vi "Create Diagnostics Addon From Configuration.vi"(7 "Merge Path (.dat)":path, 8 "error in (no error)":errorcluster, 10 "Configuration":T1 {"DID Outputs"."Frames"."Signals"."Byte Order" items=["Little Endian", "Big Endian"]; "DID Outputs"."Frames"."Signals"."Data Type" items=["Signed", "Unsigned", "IEEE Float"]; "Memory Inputs"."Frames"."Signals"."Byte Order" items=["Little Endian", "Big Endian"]; "Memory Inputs"."Frames"."Signals"."Data Type" items=["Signed", "Unsigned", "IEEE Float"]; "Memory Outputs"."Frames"."Signals"."Byte Order" items=["Little Endian", "Big Endian"]; "Memory Outputs"."Frames"."Signals"."Data Type" items=["Signed", "Unsigned", "IEEE Float"]; "Routines"."Routine Array"."Stop Parameters"."Response"."Byte Order" items=["Little Endian", "Big Endian"]; "Routines"."Routine Array"."Stop Parameters"."Response"."Data Type" items=["Signed", "Unsigned", "IEEE Float"]; "Routines"."Routine Array"."Stop Parameters"."Cmd"."Byte Order" items=["Little Endian", "Big Endian"]; "Routines"."Routine Array"."Stop Parameters"."Cmd"."Data Type" items=["Signed", "Unsigned", "IEEE Float"]; "Routines"."Routine Array"."Request Parameters"."Response"."Byte Order" items=["Little Endian", "Big Endian"]; "Routines"."Routine Array"."Request Parameters"."Response"."Data Type" items=["Signed", "Unsigned", "IEEE Float"]; "Routines"."Routine Array"."Request Parameters"."Cmd"."Byte Order" items=["Little Endian", "Big Endian"]; "Routines"."Routine Array"."Request Parameters"."Cmd"."Data Type" items=["Signed", "Unsigned", "IEEE Float"]; "Routines"."Routine Array"."Start Parameters"."Response"."Byte Order" items=["Little Endian", "Big Endian"]; "Routines"."Routine Array"."Start Parameters"."Response"."Data Type" items=["Signed", "Unsigned", "IEEE Float"]; "Routines"."Routine Array"."Start Parameters"."Cmd"."Byte Order" items=["Little Endian", "Big Endian"]; "Routines"."Routine Array"."Start Parameters"."Cmd"."Data Type" items=["Signed", "Unsigned", "IEEE Float"]; "IO Controls"."IO Control Array"."Signals"."Response"."Byte Order" items=["Little Endian", "Big Endian"]; "IO Controls"."IO Control Array"."Signals"."Response"."Data Type" items=["Signed", "Unsigned", "IEEE Float"]; "IO Controls"."IO Control Array"."Signals"."Cmd"."Byte Order" items=["Little Endian", "Big Endian"]; "IO Controls"."IO Control Array"."Signals"."Cmd"."Data Type" items=["Signed", "Unsigned", "IEEE Float"]; "DTC"."DTC Control"."Signals"."Byte Order" items=["Little Endian", "Big Endian"]; "DTC"."DTC Control"."Signals"."Data Type" items=["Signed", "Unsigned", "IEEE Float"]; "Diagnostics Basic Configuraiton"."IO Mode" items=["CAN 2.0", "CAN FD", "CAN FD+BRS"]; "Diagnostics Basic Configuraiton"."Fill Byte" format="%.0x"; "Diagnostics Basic Configuraiton"."VW TP Channel ID" format="%.0x"; "Diagnostics Basic Configuraiton"."Receive UUDT ID" format="%.0x"; "Diagnostics Basic Configuraiton"."Receive Extension" format="%.0x"; "Diagnostics Basic Configuraiton"."Transmit Extension" format="%.0x"; "Diagnostics Basic Configuraiton"."Receive ID" format="%.0x"; "Diagnostics Basic Configuraiton"."Transmit ID" format="%.0x"; "DID Inputs"."Frames"."Signals"."Byte Order" items=["Little Endian", "Big Endian"]; "DID Inputs"."Frames"."Signals"."Data Type" items=["Signed", "Unsigned", "IEEE Float"]; "PID Inputs"."Frames"."Signals"."Byte Order" items=["Little Endian", "Big Endian"]; "PID Inputs"."Frames"."Signals"."Data Type" items=["Signed", "Unsigned", "IEEE Float"]; "PID Outputs"."Frames"."Signals"."Byte Order" items=["Little Endian", "Big Endian"]; "PID Outputs"."Frames"."Signals"."Data Type" items=["Signed", "Unsigned", "IEEE Float"]}, 11 "Custom Devices Ref":refnum<k24>) -> (0 "error out":errorcluster, 3 "Custom Devices Ref":refnum<k24>)   [LabVIEW 2019, in "Diagnostics Addon SysDef API.lvlib"]
uses:
  Diagnostics Addon SysDef API.lvlib
  System Explorer/Types/SysDef.Export.ctl
  Shared/Types/CAN.ctl
  Shared/Types/CAN.Interface.ctl
  Shared/Types/Protocol.ctl
  Shared/Types/Transport.ctl
  Shared/Types/Security.ctl
  Shared/Types/Security.Type.ctl
  System Explorer/Types/Frames.Export.ctl
  System Explorer/Types/Frame.Export.ctl
  Shared/Types/Signal.ctl
  System Explorer/Types/DPIDs.Export.ctl
  System Explorer/Types/DPID.Export.ctl
  Shared/Types/DPID.ctl
  Shared/Types/DPID.Rate.ctl
  System Explorer/Types/DTC.Export.ctl
  Shared/Types/DTC.Settings.ctl
  Shared/Types/DTC.Descriptor.ctl
  System Explorer/Types/DTCControl.Export.ctl
  Shared/Types/986x.ctl
  System Explorer/Types/Command.Export.ctl
  System Explorer/Types/Status.Export.ctl
  System Explorer/Types/IOControls.Export.ctl
  System Explorer/Types/IO.Export.ctl
  System Explorer/Types/CmdResp.Export.ctl
  System Explorer/Types/Routines.Export.ctl
  System Explorer/Types/Routine.Export.ctl
  System Explorer/Types/UserDefined.Export.ctl
  System Explorer/Types/UserDefined.Group.Export.ctl
  System Explorer/Types/UserDefined.Group.Message.Export.ctl
  NationalInstruments.VeriStand.SystemDefinitionAPI
  NationalInstruments.VeriStand.SystemStorage
  Shared/SubVIs/Constants.vi
  Shared/Diagnostics Addon Shared.lvlib
  System Explorer/Diagnostics Addon System Explorer.lvlib
  <vilib>/NI/NI VeriStand Custom Device Import and Export Tool/ImportExport.lvlib
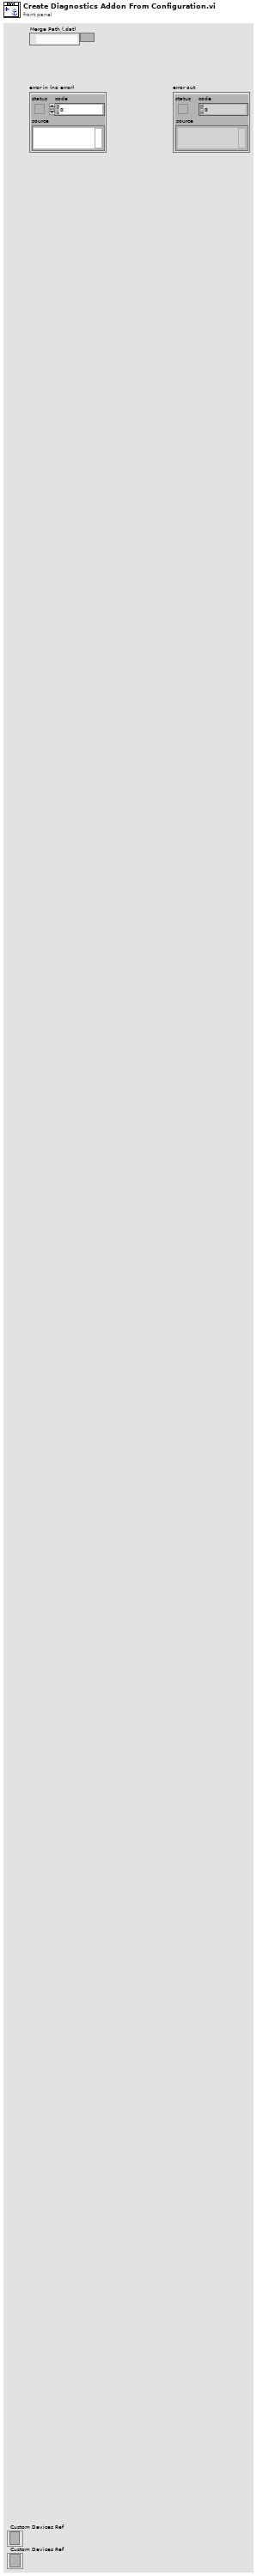
[diagram p1: front panel]
types:
  T1 = typedef "Diagnostics Addon System Explorer.lvlib/SysDef.Export.ctl" = cluster{"Name":string, "Description":string, "Diagnostics Basic Configuraiton":T2, "DID Outputs":T8, "DID Inputs":T8, "PID Outputs":T8, "PID Inputs":T8, "DPIDs":T11, "DTC":T15, "NI 986x Support":T19, "Commands":T20, "Status":T21, "IO Controls":T22, "Routines":T25, "Memory Outputs":T8, "Memory Inputs":T8, "User Defined":T27}
  T2 = typedef "Diagnostics Addon Shared.lvlib/CAN.ctl" = cluster{"Interface":T3, "Baud Rate":u64, "Diagnostic Protocol":T4, "Transport Protocol":T5, "Transmit ID":u32, "Receive ID":u32, "Transmit Extension":u8, "Receive Extension":u8, "Receive UUDT ID":u32, "Enable Stream":bool, "VW TP Channel ID":u32, "Fill Frame":bool, "Fill Byte":u8, "Termination":bool, "LIN Cluster":refnum<k21>, "NAD":u8, "IO Mode":u32, "Max DLC":u16, "FD Baud Rate":u64, "Security":T6}
  T3 = typedef "Diagnostics Addon Shared.lvlib/CAN.Interface.ctl" = string
  T4 = typedef "Diagnostics Addon Shared.lvlib/Protocol.ctl" = enum16{"GMLAN", "KWP-2000", "UDS", "User-Defined"}
  T5 = typedef "Diagnostics Addon Shared.lvlib/Transport.ctl" = enum16{"ISO TP - Normal Mode", "ISO TP - Mixed Mode", "VW TP 2.0", "Diagnostics on IP", "ISO TP LIN"}
  T6 = typedef "Diagnostics Addon Shared.lvlib/Security.ctl" = cluster{"Type":T7, "Source DLL Path":path, "Target DLL Path":path, "Security Level":u8, "Master Key":string}
  T7 = typedef "Diagnostics Addon Shared.lvlib/Security.Type.ctl" = enum16{"None", "DLL", "MasterKey"}
  T8 = typedef "Diagnostics Addon System Explorer.lvlib/Frames.Export.ctl" = cluster{"Description":string, "Frames":T9[]}
  T9 = typedef "Diagnostics Addon System Explorer.lvlib/Frame.Export.ctl" = cluster{"Name":string, "Description":string, "ID":u32, "Signals":T10[]}
  T10 = typedef "Diagnostics Addon Shared.lvlib/Signal.ctl" = cluster{"Start Bit":u32, "Length":u32, "Scaling Factor":dbl, "Scaling Offset":dbl, "Minimum":dbl, "Maximum":dbl, "Data Type":u32, "Byte Order":u32, "Default Value":dbl, "Name":string, "Units":string, "Description":string}
  T11 = typedef "Diagnostics Addon System Explorer.lvlib/DPIDs.Export.ctl" = cluster{"Description":string, "DPIDs":T12[]}
  T12 = typedef "Diagnostics Addon System Explorer.lvlib/DPID.Export.ctl" = cluster{"Name":string, "Description":string, "DPID":T13}
  T13 = typedef "Diagnostics Addon Shared.lvlib/DPID.ctl" = cluster{"DPID ID":u8, "Speed":T14, "PIDs":u16[]}
  T14 = typedef "Diagnostics Addon Shared.lvlib/DPID.Rate.ctl" = enum16{"Slow", "Medium", "Fast"}
  T15 = typedef "Diagnostics Addon System Explorer.lvlib/DTC.Export.ctl" = cluster{"Description":string, "Settings":T16, "DTC Control":T18, "Created DTCs":u32}
  T16 = typedef "Diagnostics Addon Shared.lvlib/DTC.Settings.ctl" = cluster{"Descriptor":T17, "Value.Code":dbl[], "Value.String":string[], "Value.J2012String":string[], "Status.Code":dbl[], "Status.String":string[]}
  T17 = typedef "Diagnostics Addon Shared.lvlib/DTC.Descriptor.ctl" = cluster{"DTC Byte Length":i32, "Status Byte Length":i32, "Add Data Byte Length":i32, "Byte Order":enum16{"Motorola", "Intel"}}
  T18 = typedef "Diagnostics Addon System Explorer.lvlib/DTCControl.Export.ctl" = cluster{"Description":string, "Signals":T10[]}
  T19 = typedef "Diagnostics Addon Shared.lvlib/986x.ctl" = cluster{"Enable":bool, "RIO Device":string, "Bitfile":path}
  T20 = typedef "Diagnostics Addon System Explorer.lvlib/Command.Export.ctl" = cluster{"Description":string}
  T21 = typedef "Diagnostics Addon System Explorer.lvlib/Status.Export.ctl" = cluster{"Description":string}
  T22 = typedef "Diagnostics Addon System Explorer.lvlib/IOControls.Export.ctl" = cluster{"Description":string, "IO Control Array":T23[]}
  T23 = typedef "Diagnostics Addon System Explorer.lvlib/IO.Export.ctl" = cluster{"Name":string, "Description":string, "ID":u16, "Signals":T24}
  T24 = typedef "Diagnostics Addon System Explorer.lvlib/CmdResp.Export.ctl" = cluster{"Cmd":T10[], "Response":T10[]}
  T25 = typedef "Diagnostics Addon System Explorer.lvlib/Routines.Export.ctl" = cluster{"Description":string, "Routine Array":T26[]}
  T26 = typedef "Diagnostics Addon System Explorer.lvlib/Routine.Export.ctl" = cluster{"Name":string, "Description":string, "ID":u16, "Start Parameters":T24, "Request Parameters":T24, "Stop Parameters":T24}
  T27 = typedef "Diagnostics Addon System Explorer.lvlib/UserDefined.Export.ctl" = cluster{"Description":string, "Groups":T28[]}
  T28 = typedef "Diagnostics Addon System Explorer.lvlib/UserDefined.Group.Export.ctl" = cluster{"Name":string, "Description":string, "Messages":T29[]}
  T29 = typedef "Diagnostics Addon System Explorer.lvlib/UserDefined.Group.Message.Export.ctl" = cluster{"Name":string, "Description":string, "Signals":T24}
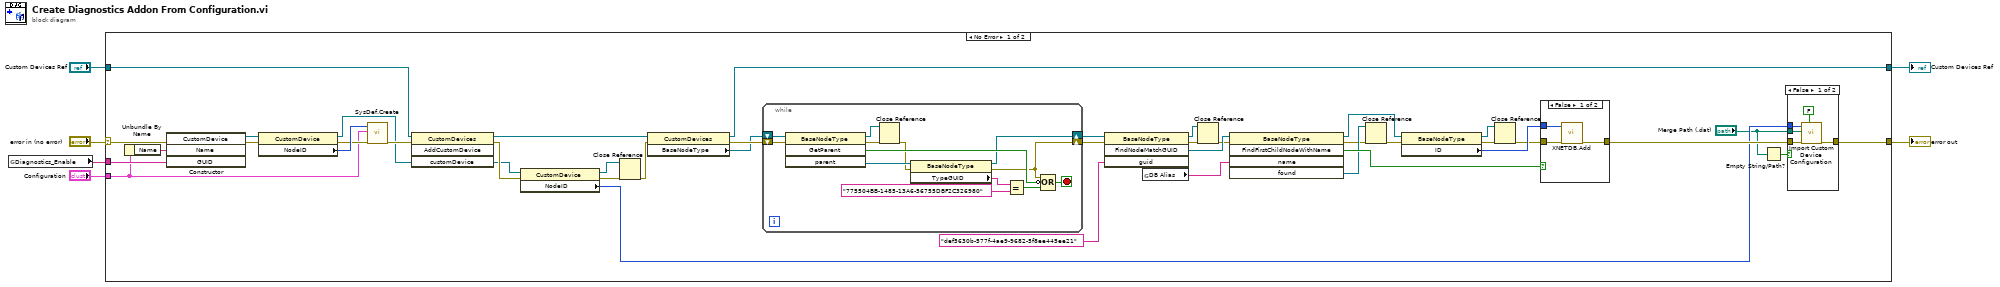
[diagram p0: block diagram]
diagram:
  n1 = global read "Constants.vi" "Diagnostics_Enable"() -> (w6:string)
  n2 = case shown="No Error" "error in (no error)" {
    selector: "error in (no error)" -> [w38 w72]
    tunnel: w6 -> [w45 _]
    tunnel: "Configuration" -> [w42 _]
    tunnel: [w15 w72] -> w4
    tunnel: "Custom Devices Ref" -> [w39 w71]
    tunnel: [w33 w71] -> w2
    frame No Error {
      n3 = Unbundle By Name(w42) -> ("Name"=w41:string)
      n4 = constructor class="CustomDevice"(error in=w38, "Name"=w41, "GUID"=w45) -> (reference out=w47:refnum<k24>, error out=w46:errorcluster)  [unwired: 2 in, 3 out]
      n5 = property class="CustomDevice"(reference=w47, error in=w46) -> (reference out=w11:refnum<k24>, error out=w43:errorcluster, "NodeID"=w44:u64)
      n6 = call "SysDef.Create.vi"("error in (no error)"=w43, "Configuration"=w42, "Device Item Ref in"=w44) -> ("error out"=w40:errorcluster)  [unwired: 7 in, 1 out]
      n7 = invoke class="CustomDevices" method="AddCustomDevice"(reference=w39, error in=w40, "customDevice"=w11) -> (reference out=w34:refnum<k24>, error out=w13:errorcluster)  [unwired: 1 in, 2 out]
      n8 = property class="CustomDevice"(reference=w11, error in=w13) -> (reference out=w10:refnum<k24>, error out=w12:errorcluster, "NodeID"=w9:u64)
      n9 = Close Reference(reference=w10, error in (no error)=w12) -> (error out=w37:errorcluster)
      n10 = property class="CustomDevices"(reference=w34, error in=w37) -> (reference out=w33:refnum<k24>, error out=w36:errorcluster, "BaseNodeType"=w35:refnum<k24>)
      n11 = while {
        shift-right: [w55] -> w30
        shift-left: w36 -> [w65]
        shift-right: [w54] -> w32
        shift-left: w35 -> [w66]
        stop <- w61 stop-if-true
        n12 = invoke class="BaseNodeType" method="GetParent"(reference=w66, error in=w65) -> (reference out=w56:refnum<k24>, error out=w58:errorcluster, "GetParent"=w62:bool, "parent"=w64:refnum<k24>)  [unwired: 2 in]
        n13 = Close Reference(reference=w56, error in (no error)=w58) -> (error out=w57:errorcluster)
        n14 = property class="BaseNodeType"(reference=w64, error in=w57) -> (reference out=w54:refnum<k24>, error out=w55:errorcluster, "TypeGUID"=w59:string)
        n15 = Equal?(x=w59, y="775504BB-1485-13A6-56755DBF2C326980") -> (x = y?=w63:bool)
        n16 = Compound Arithmetic op=OR(w55, invert w62, w63) -> (w61:bool)
      }
      n17 = invoke class="BaseNodeType" method="FindNodeMatchGUID"(reference=w32, error in=w30, "guid"="def5630b-577f-4ae9-9682-5f8ee445ee21" ("string")) -> (reference out=w29:refnum<k24>, error out=w28:errorcluster, "FindNodeMatchGUID"=w27:refnum<k24>)  [unwired: 1 in, 1 out]
      n18 = global read "Constants.vi" "DB Alias"() -> (w26:string)
      n19 = Close Reference(reference=w29, error in (no error)=w28) -> (error out=w23:errorcluster)
      n20 = invoke class="BaseNodeType" method="FindFirstChildNodeWithName"(reference=w27, error in=w23, "name"=w26) -> (reference out=w24:refnum<k24>, error out=w21:errorcluster, "FindFirstChildNodeWithName"=w25:bool, "found"=w22:refnum<k24>)  [unwired: 2 in, 1 out]
      n21 = Close Reference(reference=w22, error in (no error)=w21) -> (error out=w20:errorcluster)
      n22 = property class="BaseNodeType"(reference=w24, error in=w20) -> (reference out=w18:refnum<k24>, error out=w17:errorcluster, "ID"=w19:u64)
      n23 = Close Reference(reference=w18, error in (no error)=w17) -> (error out=w16:errorcluster)
      n24 = case shown="False" w25 {
        tunnel: [w69 w70] -> w14
        tunnel: w16 -> [w68 w70]
        tunnel: w19 -> [w67 _]
        frame False {
          n25 = call "XNETDB.Add.vi"("error in (no error)"=w68, "Databases Section Ref"=w67) -> ("error out"=w69:errorcluster)  [unwired: 9 in]
        }
        frame True {
        }
      }
      n26 = Empty String/Path?(string/path="Merge Path (.dat)") -> (empty?=w7:bool)
      n27 = case shown="False" w7 {
        tunnel: [w52 w53] -> w15
        tunnel: w14 -> [w51 w53]
        tunnel: w9 -> [w50 _]
        tunnel: "Merge Path (.dat)" -> [w49 _]
        frame False {
          n28 = call <vilib>:"Import Custom Device Configuration.vi"("Overwrite Existing?"=FALSE, "error in (no error)"=w51, "Path"=w49, "NodeID"=w50) -> ("error out"=w52:errorcluster)  [unwired: 5 in, 2 out]
        }
        frame True {
        }
      }
    }
    frame Error {
    }
  }
  "error out" <- w4
  "Custom Devices Ref" <- w2
